vi "Size.vi"(8 "error in (no error)":errorcluster, 11 "Vector Parent in":refnum<class "Vector Parent.lvclass">) -> (0 "error out":errorcluster, 2 "size":i32, 3 "Vector Parent out":refnum<class "Vector Parent.lvclass">)   [LabVIEW 2021, in "Vector Parent.lvclass"]
uses:
  Vector Parent.lvclass
  Vector Parent.lvclass/Vector Parent.ctl
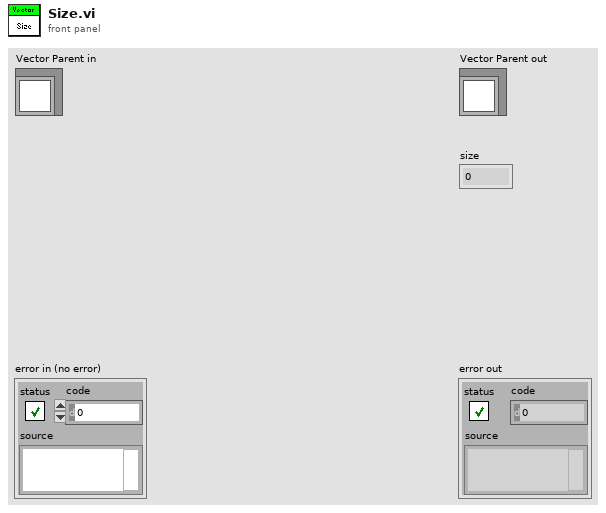
[diagram p1: front panel]
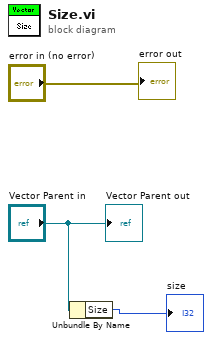
[diagram p0: block diagram]
diagram:
  n1 = Unbundle By Name("Vector Parent in") -> ("Size"=→"size":u32)
  "error out" <- "error in (no error)"
  "Vector Parent out" <- "Vector Parent in"
